vi "Add to Project.vi"(8 "error in (no error)":errorcluster, 11 "QControl Creation in":refnum<class "QControl Creation.lvclass">) -> (0 "error out":errorcluster, 3 "QControl Creation (dup)":refnum<class "QControl Creation.lvclass">)   [LabVIEW 2015, in "QControl Creation.lvclass"]
doc: "<b> </b> <b> </b>\n©2016 Q Software Innovations, LLC (QSI)\nwritten by Quentin Alldredge\nproduced in LabVIEW 2015\n\nsupport@qsoftwareinnovations.com\nwww.qsoftwareinnovations.com\n\nAll rights reserved.\n\nRedistribution and use in source and binary forms, with or without modification, are permitted provided that the following conditions are met:\n\n * Redistributions of source code must retain the above copyright notice, this list of conditions and the following disclaimer.\n * Redistributions in binary form must reproduce the above copyright notice, this list of conditions and the following disclaimer in the documentation and/or other materials provided with the distribution.\n * Neither the name of Q Software Innovations, LLC. nor the names of its contributors may be used to endorse or promote products derived from this software without specific prior written permission.\n\nTHIS SOFTWARE IS PROVIDED BY THE COPYRIGHT HOLDERS AND CONTRIBUTORS \"AS IS\" AND ANY EXPRESS OR IMPLIED WARRANTIES, INCLUDING, BUT NOT LIMITED TO, THE IMPLIED WARRANTIES OF MERCHANTABILITY AND FITNESS FOR A PARTICULAR PURPOSE ARE DISCLAIMED. IN NO EVENT SHALL THE COPYRIGHT OWNER OR CONTRIBUTORS BE LIABLE FOR ANY DIRECT, INDIRECT, INCIDENTAL, SPECIAL, EXEMPLARY, OR CONSEQUENTIAL DAMAGES (INCLUDING, BUT NOT LIMITED TO, PROCUREMENT OF SUBSTITUTE GOODS OR SERVICES; LOSS OF USE, DATA, OR PROFITS; OR BUSINESS INTERRUPTION) HOWEVER CAUSED AND ON ANY THEORY OF LIABILITY, WHETHER IN CONTRACT, STRICT LIABILITY, OR TORT (INCLUDING NEGLIGENCE OR OTHERWISE) ARISING IN ANY WAY OUT OF THE USE OF THIS SOFTWARE, EVEN IF ADVISED OF THE POSSIBILITY OF SUCH DAMAGE."
uses:
  QControl Creation.lvclass
  QControl Creation.lvclass/QControl Creation.ctl
  New QControl Info/New QControl Info.lvclass/New QControl Info.ctl
  New QControl Info/Read Target Ref.vi
  New QControl Info/Read New Class Path.vi
  New QControl Info/Read App Refnum.vi
  New QControl Info/Read ProjectItem Ref.vi
  New QControl Info/Read Add to Location.vi
  <vilib>/Utility/error.llb/Error Cluster From Error Code.vi
  <vilib>/ErrorRing/Error Ring.xnode
  New QControl Info/New QControl Info.lvclass
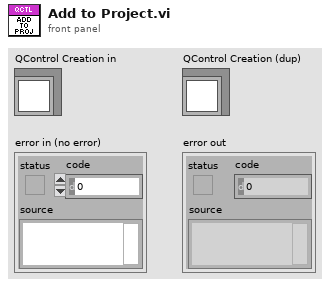
[diagram p1: front panel]
types:
  T1 = enum16{"Don't Add", "To Target", "To Project Item"}
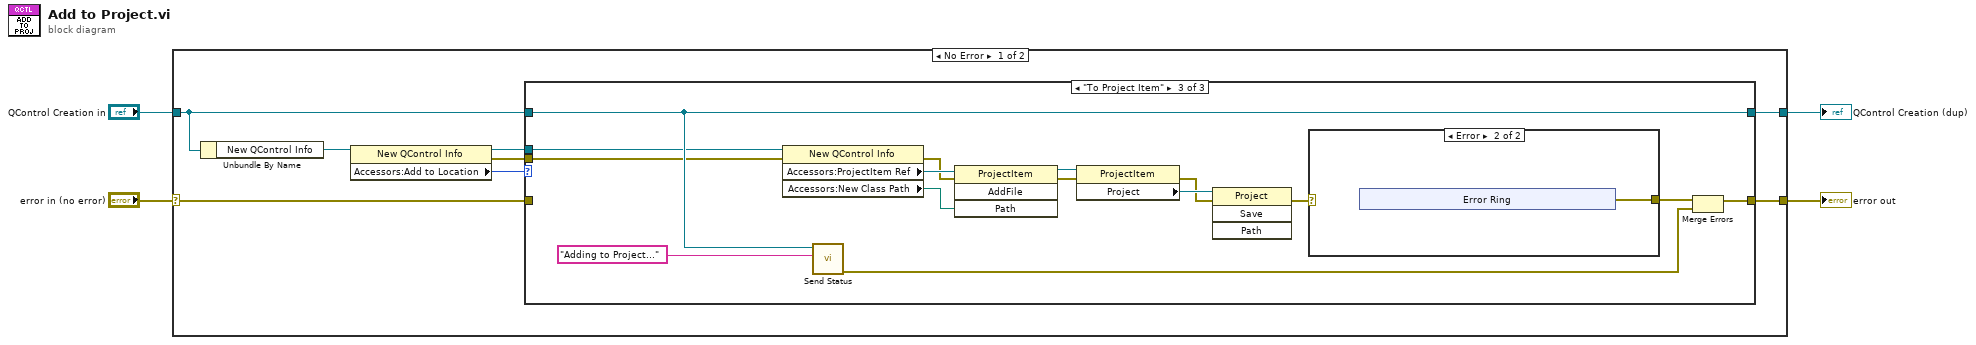
[diagram p0: block diagram]
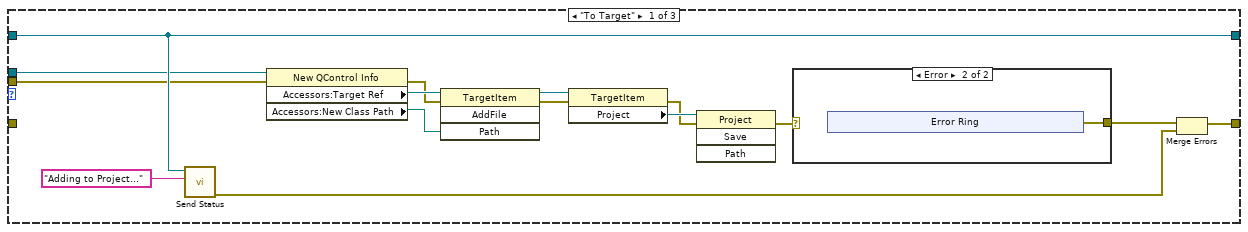
[diagram p2: hidden frame]
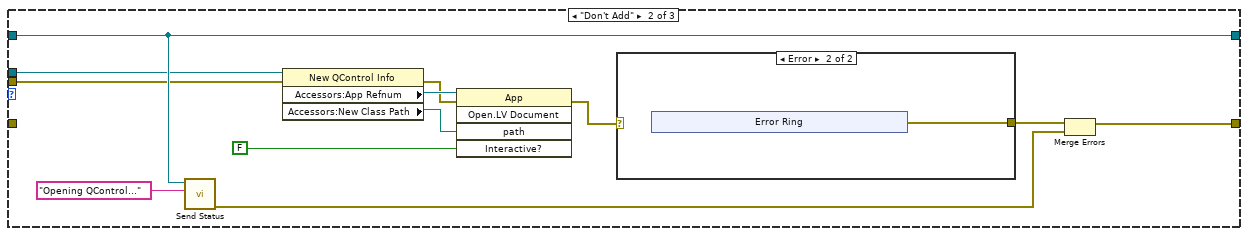
[diagram p4: hidden frame]
diagram:
  n1 = case shown="No Error" "error in (no error)" {
    selector: "error in (no error)" -> [w8 w77]
    tunnel: [w9 w77] -> w3
    tunnel: [w11 w76] -> w1
    tunnel: "QControl Creation in" -> [w10 w76]
    frame No Error {
      n2 = Unbundle By Name(w10) -> ("New QControl Info"=w12:refnum<data-value>)
      n3 = property class="New QControl Info"(reference=w12) -> (reference out=w6:refnum<data-value>, error out=w5:errorcluster, "Accessors:Add to Location"=w7:T1)  [unwired: 1 in]
      n4 = case shown="\"To Project Item\"" w7 {
        tunnel: [w22 w44 w63] -> w11
        tunnel: w10 -> [w22 w44 w63]
        tunnel: [w19 w43 w62] -> w9
        tunnel: w8 -> [_ _ _]
        tunnel: w6 -> [w17 w39 w58]
        tunnel: w5 -> [w16 w36 w57]
        frame "To Target" {
          n5 = call "Send Status.vi"("Status"="Adding to Project..." ("Add Item"), "QControl Creation in"=w22) -> ("error out (dup)"=w18:errorcluster)  [unwired: 8 in, 1 out]
          n6 = property class="New QControl Info"(reference=w17, error in=w16) -> (error out=w13:errorcluster, "Accessors:Target Ref"=w15:refnum<vi>, "Accessors:New Class Path"=w14:path)  [unwired: 1 out]
          n7 = invoke class="TargetItem" method="AddFile"(reference=w15, error in=w13, "Path"=w14) -> (reference out=w27:refnum<vi>, error out=w26:errorcluster)  [unwired: 1 in, 2 out]
          n8 = property class="TargetItem"(reference=w27, error in=w26) -> (error out=w24:errorcluster, "Project"=w25:refnum<vi>)  [unwired: 1 out]
          n9 = invoke class="Project" method="Save"(reference=w25, error in=w24) -> (error out=w21:errorcluster)  [unwired: 2 in, 3 out]
          n10 = case shown="Error" w21 {
            selector: w21 -> [w28 _]
            tunnel: [w28 w29] -> w20
            frame No Error {
            }
            frame Error {
              n11 = xnode "Error Ring"() -> ("error out"=w29:errorcluster)
            }
          }
          n12 = Merge Errors(w20, w18) -> (w19:errorcluster)
        }
        frame "Don't Add" {
          n13 = call "Send Status.vi"("Status"="Opening QControl..." ("Add Item"), "QControl Creation in"=w44) -> ("error out (dup)"=w42:errorcluster)  [unwired: 8 in, 1 out]
          n14 = property class="New QControl Info"(reference=w39, error in=w36) -> (error out=w35:errorcluster, "Accessors:App Refnum"=w38:refnum<vi>, "Accessors:New Class Path"=w37:path)  [unwired: 1 out]
          n15 = invoke class="App" method="Open.LV Document"(reference=w38, error in=w35, "path"=w37, "Interactive?"=FALSE) -> (error out=w41:errorcluster)  [unwired: 1 in, 4 out]
          n16 = case shown="Error" w41 {
            selector: w41 -> [w47 _]
            tunnel: [w47 w48] -> w40
            frame No Error {
            }
            frame Error {
              n17 = xnode "Error Ring"() -> ("error out"=w48:errorcluster)
            }
          }
          n18 = Merge Errors(w40, w42) -> (w43:errorcluster)
        }
        frame "To Project Item" {
          n19 = property class="New QControl Info"(reference=w58, error in=w57) -> (error out=w54:errorcluster, "Accessors:ProjectItem Ref"=w56:refnum<vi>, "Accessors:New Class Path"=w55:path)  [unwired: 1 out]
          n20 = call "Send Status.vi"("Status"="Adding to Project..." ("Add Item"), "QControl Creation in"=w63) -> ("error out (dup)"=w61:errorcluster)  [unwired: 8 in, 1 out]
          n21 = invoke class="ProjectItem" method="AddFile"(reference=w56, error in=w54, "Path"=w55) -> (reference out=w68:refnum<vi>, error out=w67:errorcluster)  [unwired: 1 in, 2 out]
          n22 = property class="ProjectItem"(reference=w68, error in=w67) -> (error out=w65:errorcluster, "Project"=w66:refnum<vi>)  [unwired: 1 out]
          n23 = invoke class="Project" method="Save"(reference=w66, error in=w65) -> (error out=w59:errorcluster)  [unwired: 2 in, 3 out]
          n24 = case shown="Error" w59 {
            selector: w59 -> [w69 _]
            tunnel: [w69 w70] -> w60
            frame No Error {
            }
            frame Error {
              n25 = xnode "Error Ring"() -> ("error out"=w70:errorcluster)
            }
          }
          n26 = Merge Errors(w60, w61) -> (w62:errorcluster)
        }
      }
    }
    frame Error {
    }
  }
  "error out" <- w3
  "QControl Creation (dup)" <- w1
